vi "GetAppData.vi"(8 "Error In":errorcluster[](array[cluster]), 10 "arg":string, 11 "Bus in":refnum<class "Bus.lvclass">) -> (0 "Error Out":errorcluster[](array[cluster]), 2 "XmlData":string, 3 "Bus out":refnum<class "Bus.lvclass">)   [LabVIEW 2017, in "Bus_class.lvlib" / "Bus.lvclass"]
uses:
  Bus.lvclass
  Bus.lvclass/Bus.ctl
  Modules/AppModule/PublicAPI/Arguments/Broadcasts/clErrorRpt.ctl
  <vilib>/Utility/error.llb/Error Cluster From Error Code.vi
  <vilib>/ErrorRing/Error Ring.xnode
  TestAutomation/LTA/LTA.lvlib
  <userlib>/NIST/NISTErrorLib/NISTErrorLib.lvlib
  Modules/AppModule/AppModule.lvlib
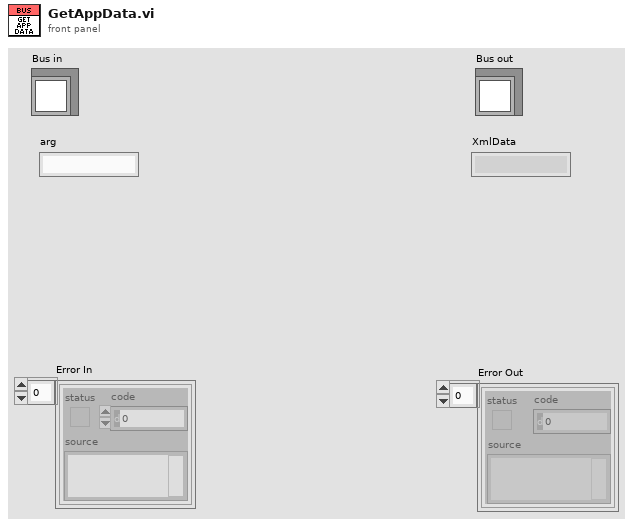
[diagram p1: front panel]
types:
  T1 = typedef "AppModule.lvlib/clErrorRpt.ctl" = cluster{"error":errorcluster, "AdditionalInfo":string}
  T2 = typedef "AppModule.lvlib/clBroadcastEvents.ctl" = cluster{"DidInit":refnum<user-event>, "StatusUpdate":refnum<user-event>, "ErrorReport":refnum<user-event>, "DidStop":refnum<user-event>, "PathToINI":refnum<user-event>, "InputData":refnum<user-event>, "OutputData":refnum<user-event>, "BcAppInfo":refnum<user-event>, "ConfigData":refnum<user-event>}
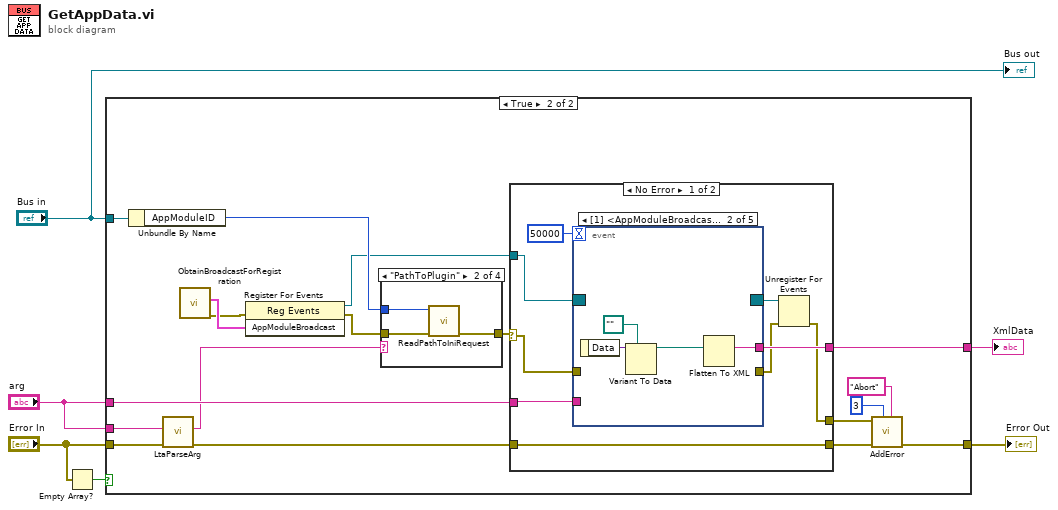
[diagram p0: block diagram]
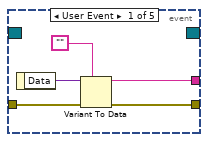
[diagram p3: hidden frame]
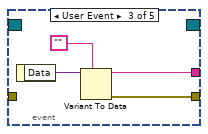
[diagram p4: hidden frame]
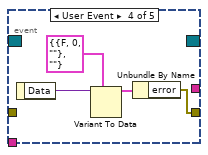
[diagram p5: hidden frame]
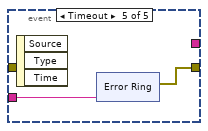
[diagram p6: hidden frame]
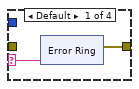
[diagram p8: hidden frame]
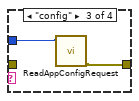
[diagram p9: hidden frame]
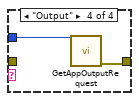
[diagram p10: hidden frame]
diagram:
  n1 = Empty Array?(array="Error In") -> (empty?=w6:bool)
  n2 = case shown="True" w6 {
    tunnel: "Bus in" -> [_ w21]
    tunnel: "Error In" -> [w7 w25]
    tunnel: [w7 w22] -> w4
    tunnel: "arg" -> [_ w24]
    tunnel: "arg" -> [_ w20]
    tunnel: [_ w19] -> w2
    frame False {
    }
    frame True {
      n3 = Unbundle By Name(w21) -> ("AppModuleID"=w13:i32)
      n4 = call "LtaParseArg.vi"("Error In"=w25, "Arg In"=w24) -> ("Error Out"=w23:errorcluster[], "Arg 1"=w12:string)  [unwired: 6 in, 2 out]
      n5 = call "ObtainBroadcastForRegistration.vi"() -> ("error out"=w8:errorcluster, "AppModuleBroadcast"=w9:T2)  [unwired: 10 in]
      n6 = register-events(error in=w8, w9) -> (reference out=w11:refnum<event-registration>, error out=w10:errorcluster)  [unwired: 1 in]
      n7 = case shown="\"PathToPlugin\"" w12 {
        selector: w12 -> [w63 _ _ _]
        tunnel: [w64 w73 w75 w78] -> w18
        tunnel: w13 -> [_ w74 w76 w77]
        tunnel: w10 -> [_ w72 _ _]
        frame Default {
          n8 = xnode "Error Ring"("parameter 0"=w63) -> ("error out"=w64:errorcluster)
        }
        frame "PathToPlugin" {
          n9 = call "ReadPathToIniRequest.vi"("error in (no error)"=w72, "ModuleID"=w74) -> ("error out"=w73:errorcluster)  [unwired: 9 in]
        }
        frame "config" {
          n10 = call "ReadAppConfigRequest.vi"("ModuleID"=w76) -> ("error out"=w75:errorcluster)  [unwired: 10 in]
        }
        frame "Output" {
          n11 = call "GetAppOutputRequest.vi"("ModuleID"=w77) -> ("error out"=w78:errorcluster)  [unwired: 10 in]
        }
      }
      n12 = case shown="No Error" w18 {
        selector: w18 -> [w26 w62]
        tunnel: w23 -> [w31 w61]
        tunnel: [w28 w62] -> w17
        tunnel: [w31 w61] -> w16
        tunnel: w20 -> [w34 _]
        tunnel: [w32 _] -> w19
        tunnel: w11 -> [w27 _]
        frame No Error {
          n13 = event shown="[1] <AppModuleBroadcast.PathToINI>: User Event" {
            selector: w27 -> [_ _ _ _ _]
            dyn-events: [_ _ _ _ _] -> w30
            timeout: 50000 -> [_ _ _ _ _]
            tunnel: [w38 _ w46 w49 w53] -> w29
            tunnel: w34 -> [_ _ _ _ w52]
            tunnel: [w36 w41 w45 _ _] -> w32
            tunnel: w26 -> [w35 _ _ _ _]
            event User Event {
              n14 = event-data() -> ("Data"=w39:variant)  [unwired: 1 in]
              n15 = Variant To Data(error in=w35, type="", Variant=w39) -> (data=w36:string, error out=w38:errorcluster)
            }
            event User Event {
              n16 = event-data() -> ("Data"=w43:variant)  [unwired: 1 in]
              n17 = Variant To Data(type=path "", Variant=w43) -> (data=w40:path)  [unwired: 1 in, 1 out]
              n18 = Flatten To XML(anything=w40) -> (xml string=w41:string)
            }
            event User Event {
              n19 = event-data() -> ("Data"=w47:variant)  [unwired: 1 in]
              n20 = Variant To Data(type="", Variant=w47) -> (data=w45:string, error out=w46:errorcluster)  [unwired: 1 in]
            }
            event User Event {
              n21 = event-data() -> ("Data"=w50:variant)  [unwired: 1 in]
              n22 = Variant To Data(type=T1 {"error"={"status"=FALSE, "code"=0, "source"=""}, "AdditionalInfo"=""} ("Cluster"), Variant=w50) -> (data=w51:T1)  [unwired: 1 in, 1 out]
              n23 = Unbundle By Name(w51) -> ("error"=w49:errorcluster)
            }
            event Timeout {
              n24 = event-data() -> ()  [unwired: 1 in, 3 out]
              n25 = xnode "Error Ring"("parameter 0"=w52) -> ("error out"=w53:errorcluster)
            }
          }
          n26 = Unregister For Events(event registration refnum=w30, error in=w29) -> (error out=w28:errorcluster)
        }
        frame Error {
        }
      }
      n27 = call <userlib>:"AddError.vi"("Severity"="Abort", "Priority"=u8 3, "ErrorArray"=w16, "error in (no error)"=w17) -> ("ErrorArray"=w22:errorcluster[])  [unwired: 6 in, 1 out]
    }
  }
  "Error Out" <- w4
  "XmlData" <- w2
  "Bus out" <- "Bus in"
